vi "rose.vi"() -> ()   [LabVIEW 2021]
uses:
  <vilib>/picture/3D Picture Control/Object/Create Object (name).vi
  <vilib>/picture/3D Picture Control/NI_3D Picture Control.lvlib
panel:
  in  "stop":bool
  out "3D Picture":refnum<vi>(3d-picture)
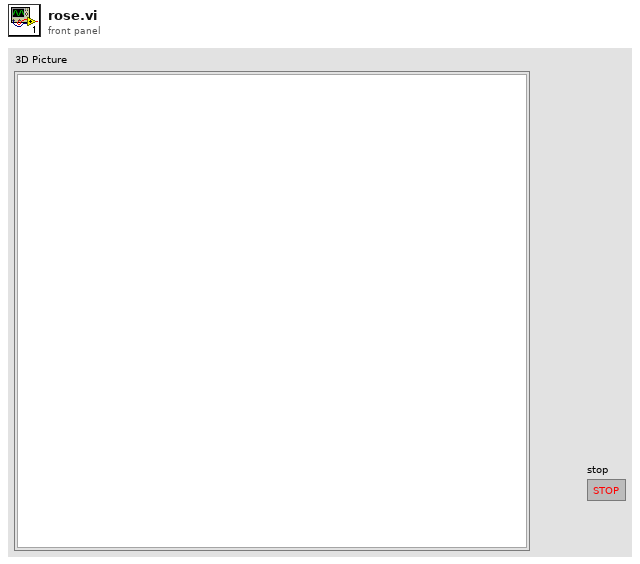
[diagram p1: front panel]
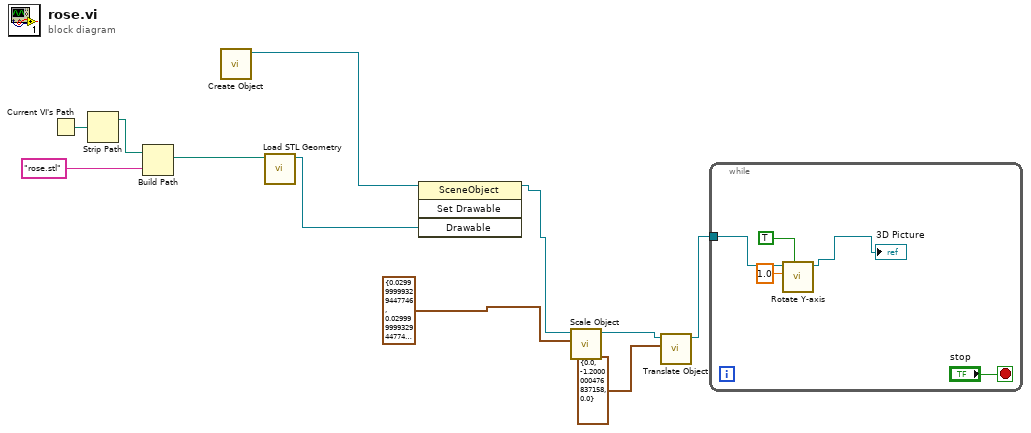
[diagram p0: block diagram]
diagram:
  n1 = Current VI's Path() -> (path=w9:path)
  n2 = Strip Path(path=w9) -> (stripped path=w10:path)  [unwired: 1 out]
  n3 = Build Path(base path=w10, name or relative path="rose.stl") -> (appended path=w8:path)
  n4 = call-poly <vilib>:"Create Object.vi"() -> ("Scene:New Object"=w7:refnum<vi>)  [unwired: 10 in, 1 out]
  n5 = call <vilib>:"Load STL Geometry.vi"("Model File"=w8) -> ("New Mesh Refnum"=w4:refnum<vi>)  [unwired: 9 in, 1 out]
  n6 = invoke class="SceneObject" method="Set Drawable"(reference=w7, "Drawable"=w4) -> (reference out=w6:refnum<vi>)  [unwired: 2 in, 3 out]
  n7 = call <vilib>:"Scale Object.vi"("Scale"=cluster{"X":sgl, "Y":sgl, "Z":sgl} {"X"=0.03, "Y"=0.03, "Z"=0.03}, "Scene.Object In"=w6) -> ("Scene.Object Out"=w3:refnum<vi>)  [unwired: 8 in, 1 out]
  n8 = call <vilib>:"Translate Object.vi"("Translation"=cluster{"X":sgl, "Y":sgl, "Z":sgl} {"X"=0.0, "Y"=-1.2, "Z"=0.0}, "Scene.Object In"=w3) -> ("Scene.Object Out"=w1:refnum<vi>)  [unwired: 8 in, 1 out]
  n9 = while {
    tunnel: w1 -> [w16]
    stop <- "stop" stop-if-true
    n10 = call <vilib>:"Rotate Y-axis.vi"("Relative?"=TRUE, "angle"=1.0, "Scene Object In"=w16) -> ("Scene Object Out"=→"3D Picture":refnum<vi>)  [unwired: 7 in, 1 out]
  }
